vi "Initialize.vi"(8 "error in (no error)":errorcluster, 11 "DAQ Class in":refnum<class "DAQ Class.lvclass">) -> (0 "error out":errorcluster, 3 "DAQ Class out":refnum<class "DAQ Class.lvclass">)   [LabVIEW 2015, in "DAQ Class.lvclass"]
uses:
  DAQ Class.lvclass
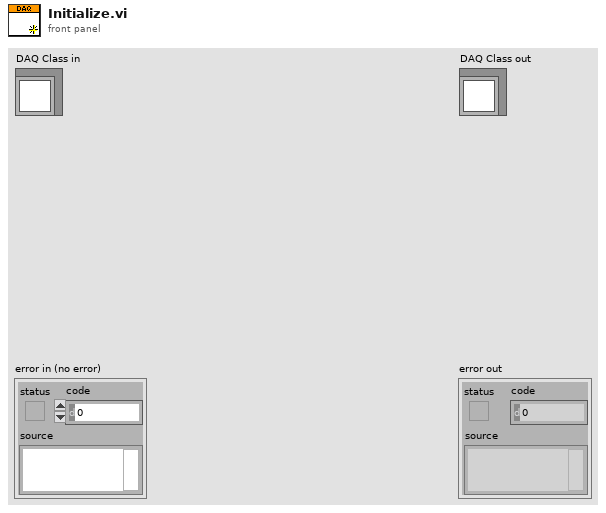
[diagram p1: front panel]
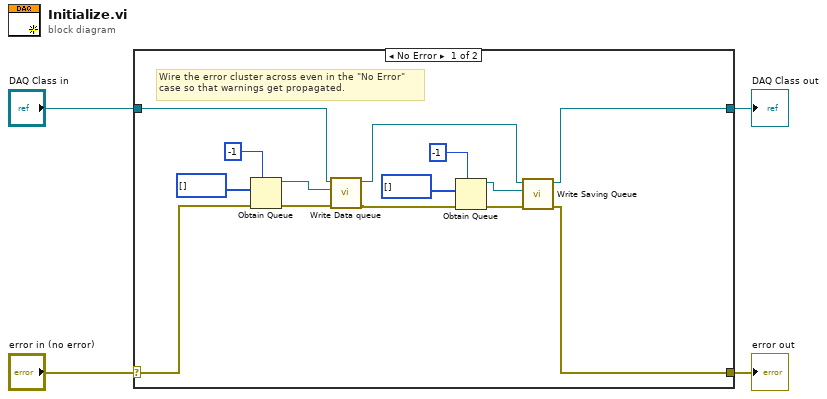
[diagram p0: block diagram]
diagram:
  n1 = case shown="No Error" "error in (no error)" {
    selector: "error in (no error)" -> [w15 w20]
    tunnel: [w7 w20] -> w3
    tunnel: [w6 w19] -> w1
    tunnel: "DAQ Class in" -> [w17 w19]
    frame No Error {
      # "Wire the error cluster across even in the \"No Error\"\ncase so that warnings get propagated."
      n2 = Obtain Queue(max queue size (-1, unlimited)=-1, element data type=u16[] [], error in (no error)=w15) -> (queue out=w18:refnum<queue>, error out=w13:errorcluster)  [unwired: 2 in, 1 out]
      n3 = call-dynamic "Write Data queue.vi"("error in (no error)"=w13, "Data queue"=w18, "DAQ Class in"=w17) -> ("error out"=w10:errorcluster, "DAQ Class out"=w5:refnum<class "DAQ Class.lvclass">)  [unwired: 7 in]
      n4 = Obtain Queue(max queue size (-1, unlimited)=-1, element data type=u16[] [], error in (no error)=w10) -> (queue out=w9:refnum<queue>, error out=w8:errorcluster)  [unwired: 2 in, 1 out]
      n5 = call-dynamic "Write Saving Queue.vi"("error in (no error)"=w8, "Saving Queue"=w9, "DAQ Class in"=w5) -> ("error out"=w7:errorcluster, "DAQ Class out"=w6:refnum<class "DAQ Class.lvclass">)  [unwired: 7 in]
    }
    frame Error {
    }
  }
  "error out" <- w3
  "DAQ Class out" <- w1
